vi "Optimize Extended Rosenbrock.vi"() -> ()   [LabVIEW 2016]
doc: "This VI shows an example of using the Unconstrained Optimization VI. The VI uses the Extended Rosenbrock Function VI to create an objective function. The VI then passes this function to the Unconstrained Optimization VI."
uses:
  <vilib>/Math Plots/3D Math Plots/3D Surface/3D Surface XCtrl/3D Surface.xctl
  <vilib>/Math Plots/3D Math Plots/3D Plot/3D Plot/Typedef/Color Ramp Cluster.ctl
  <vilib>/Analysis/1siggen.llb/Ramp Pattern by Samples.vi
  <vilib>/Math Plots/3D Math Plots/3D Surface/3D Surface Datatype/Public/Plot Helper (Vector).vi
  <vilib>/gmath/NumericalOptimization/Quasi Newton.vi
  <vilib>/gmath/NumericalOptimization/Conjugate Gradient.vi
  <vilib>/gmath/NumericalOptimization/Downhill Simplex.vi
  <vilib>/gmath/NI_Gmath.lvlib
  <vilib>/Analysis/NI_AALBase.lvlib
  <vilib>/Math Plots/3D Math Plots/3D Surface/3D Surface Datatype/3D Surface Datatype.lvclass
  <vilib>/Math Plots/3D Math Plots/3D Plot/3D Plot/3D Plot.lvclass
panel:
  in  "Conjugate gradient settings":T1={"gradient method"=enum."Polak-Ribiere", "line minimization"=enum."with derivatives"}
  in  "Stopping criteria":T2={"function tolerance"=1e-08, "parameter tolerance"=1e-10, "max iterations"=10000, "max function calls"=10000, "gradient tolerance"=-1.0, "max time (sec)"=-1.0}
  in  "Optimization Method":T3(ring)
  in  "Animate solution?":bool=TRUE
  out "Intensity Graph":dbl[][](graph)
  out "3D Surface":refnum<class "3D Plot Datatype.lvclass">[](xcontrol)
  out "Number of function evaluations":i32
  out "Minimum Value":dbl
  out "Minimum":dbl[](array[numeric])
  in  "Start":dbl[](array[numeric])=[-1.2, 2.0]
  # "Overview: Demonstrates the use of the Unconstrained Optimization VI.\nRequirements: LabVIEW Full Development System\nInstructions:\n1. Select an Optimization Method and Start position of the optimization.\n2. Run the VI and, if you have Animate Solution? set to TRUE, you can see the path of the solver on the Intensity Graph. If the solver can find the solution, you would be able to see the minimum at [1,1]. Try to run the VI again with Animate Solution? set to FALSE to observe the speed of the algorithm.\n3. Add two more points to the Start array making [-1.2, 2, -1.2, 2]. Although the graph will only show the first two variables, the Minimum array will show more points, all at 1."
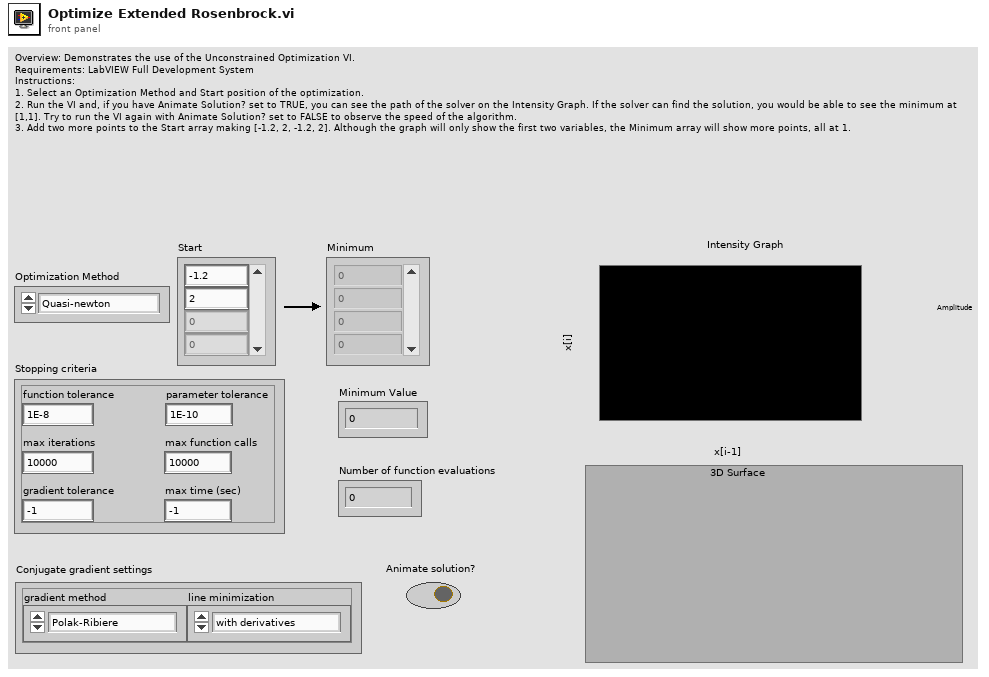
[diagram p1: front panel]
types:
  T1 = cluster{"gradient method":enum16{"Fletcher-Reeves", "Polak-Ribiere"}, "line minimization":enum16{"without derivatives", "with derivatives"}}
  T2 = cluster{"function tolerance":dbl, "parameter tolerance":dbl, "max iterations":i32, "max function calls":i32, "gradient tolerance":dbl, "max time (sec)":dbl}
  T3 = enum16{"Quasi-newton", "Conjugate Gradient", "Downhill Simplex"}
  T4 = enum16{"None", "Shaded", "Color spectrum", "Grey scale", "Custom"}
  T5 = typedef "3D Plot.lvclass/Color Ramp Cluster.ctl" = cluster{"Color Ramp Style":enum16{"None", "Shaded", "Color spectrum", "Grey scale", "Custom"}, "Color Ramp Array":u32[], "Color Ramp Index":i32[], "Interpolate?":bool, "Logarithm?":bool}
  T6 = cluster{"c":dbl, "Intensity Graph":refnum<vi>, "animate?":bool}
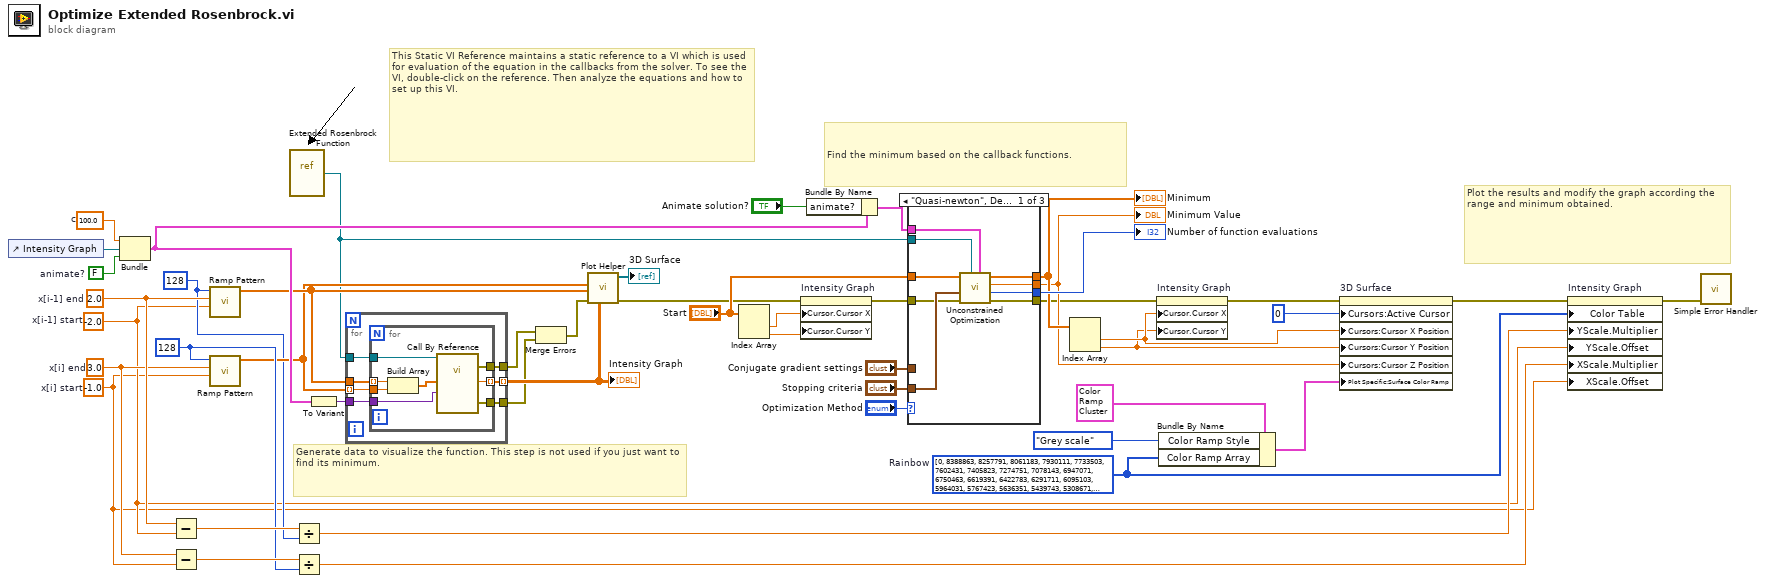
[diagram p0: block diagram]
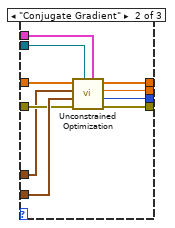
[diagram p2: hidden frame]
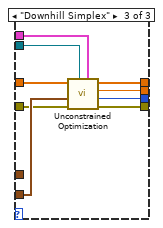
[diagram p3: hidden frame]
diagram:
  w33 = 100.0  # c
  w18 = 128 ("samples")
  w32 = FALSE  # animate?
  w41 = u32[] [0, 8388863, 8257791, 8061183, 7930111, 7733503, 7602431, 7405823, 7274751, 7078143, 6947071, 6750463, 6619391, 6422783, 6291711, 6095103, 5964031, 5767423, 5636351, 5439743, 5308671, 5112063, 4980991, 4784383, 4653311, 4456703, 4325631, 4129023, 3932415, 3801343, 3604735, 3473663, 3277055, 3145983, 2949375, 2818303, 2621695, 2490623, 2294015, 2162943, 1966335, 1835263, 1638655, 1507583, 1310975, 1179903, 983295, 852223, 655615, 524543, 327935, 196863, 511, 1791, 3071, 4351, 5631, 6911, 8191, 9471, 10751, 12031, 13311, 14591, 15871, 17151, 18431, 19711, 20991, 22271, 23551, 24831, 26111, 27391, 28671, 29951, 31231, 32511, 33791, 35071, 36351, 37631, 38911, 40191, 41471, 42751, 44031, 45311, 46591, 47871, 49151, 50431, 51711, 52991, 54271, 55551, 56831, 58111, 59391, 60671, 61951, 63231, 64511, 65532, 65527, 65522, 65517, 65512, 65507, 65502, 65497, 65492, 65487, 65482, 65477, 65472, 65467, 65462, 65457, 65452, 65447, 65442, 65437, 65432, 65427, 65422, 65417, 65412, 65407, 65402, 65397, 65392, 65387, 65382, 65377, 65372, 65367, 65362, 65357, 65352, 65347, 65342, 65337, 65332, 65327, 65322, 65317, 65312, 65307, 65302, 65297, 65292, 65287, 65282, 261888, 589568, 917248, 1244928, 1572608, 1900288, 2227968, 2555648, 2883328, 3211008, 3538688, 3866368, 4194048, 4521728, 4849408, 5177088, 5504768, 5832448, 6160128, 6487808, 6815488, 7143168, 7470848, 7798528, 8126208, 8453888, 8781568, 9109248, 9436928, 9764608, 10092288, 10419968, 10747648, 11075328, 11403008, 11730688, 12058368, 12386048, 12713728, 13041408, 13369088, 13696768, 14024448, 14352128, 14679808, 15007488, 15335168, 15662848, 15990528, 16318208, 16645888, 16775936, 16774656, 16773376, 16772096, 16770816, 16769536, 16768256, 16766976, 16765696, 16764416, 16763136, 16761856, 16760576, 16759296, 16758016, 16756736, 16755456, 16754176, 16752896, 16751616, 16750336, 16749056, 16747776, 16746496, 16745216, 16743936, 16742656, 16741376, 16740096, 16738816, 16737536, 16736256, 16734976, 16733696, 16732416, 16731136, 16729856, 16728576, 16727296, 16726016, 16724736, 16723456, 16722176, 16720896, 16719616, 16718336, 16717056, 16715776, 16714496, 16713216, 16711680]  # Rainbow
  w12 = 128 ("samples")
  w11 = -2.0  # x[i-1] start
  w39 = 2.0  # x[i-1] end
  w10 = -1.0  # x[i] start
  w36 = 3.0  # x[i] end
  # "Plot the results and modify the graph according the range and minimum obtained."
  # "Find the minimum based on the callback functions."
  # "Generate data to visualize the function. This step is not used if you just want to find its minimum."
  # "This Static VI Reference maintains a static reference to a VI which is used for evaluation of the equation in the callbacks from the solver. To see the VI, double-click on the reference. Then analyze the equations and how to set up this VI."
  n1 = control-ref of="Intensity Graph"() -> (w34:refnum<vi>)
  n2 = Bundle("c"=w33, "Intensity Graph"=w34, "animate?"=w32) -> (w31:T6)  [unwired: 1 in]
  n3 = Subtract(x=w39, y=w11) -> (x-y=w38:dbl)
  n4 = Subtract(x=w36, y=w10) -> (x-y=w37:dbl)
  n5 = call-poly <vilib>:"Ramp Pattern.vi"("start"=w11, "end"=w39, "samples"=w12) -> ("Ramp Pattern"=w19:dbl[])  [unwired: 7 in, 1 out]
  n6 = call-poly <vilib>:"Ramp Pattern.vi"("start"=w10, "end"=w36, "samples"=w18) -> ("Ramp Pattern"=w17:dbl[])  [unwired: 7 in, 1 out]
  n7 = vi-ref "Extended Rosenbrock Function.vi"() -> (w15:refnum<vi>)
  n8 = Divide(x=w38, y=w12) -> (x/y=w40:dbl)
  n9 = Divide(x=w37, y=w18) -> (x/y=w13:dbl)
  n10 = To Variant(anything=w31) -> (Variant=w44:variant)
  n11 = for {
    tunnel: [w54] -> w24 mode=indexing
    tunnel: w19 -> [w53]
    tunnel: w17 -> [w52] mode=indexing
    tunnel: w44 -> [w51]
    tunnel: [w50] -> w2
    tunnel: w15 -> [w49]
    tunnel: [w48] -> w3
    n12 = for {
      tunnel: [w62] -> w54 mode=indexing
      tunnel: w53 -> [w58] mode=indexing
      tunnel: w52 -> [w59]
      tunnel: w51 -> [w60]
      tunnel: [w57] -> w50
      tunnel: w49 -> [w56]
      tunnel: [w55] -> w48
      n13 = Build Array(w58, w59) -> (w61:dbl[])
      n14 = call-by-ref "?"(reference=w56, "data"=w60, "X"=w61) -> (error out=w55:errorcluster, 0:"error out"=w57:errorcluster, "f(X)"=w62:dbl)  [unwired: 2 in, 2 out]
    }
  }
  "Intensity Graph" <- w24
  n15 = Merge Errors(w3, w2) -> (w1:errorcluster)
  n16 = call-poly <vilib>:"Plot Helper.vi"("z matrix"=w24, "error in (no error)"=w1, "y vector"=w19, "x vector"=w17) -> ("error out"=w5:errorcluster, "3D Plot lvclass Array out"=→"3D Surface":refnum<class "3D Plot Datatype.lvclass">[])  [unwired: 2 in, 4 out]
  n17 = Index Array(array="Start") -> (element #1=w7:dbl, element #2=w6:dbl)  [unwired: 2 in]
  n18 = property on="Intensity Graph" class="IntGraph (strict)"(error in=w5, "Cursor.Cursor X"=w7, "Cursor.Cursor Y"=w6) -> (error out=w4:errorcluster)  [unwired: 1 in, 1 out]
  n19 = Bundle By Name(cluster=w31, "animate?"="Animate solution?") -> (w30:T6)
  n20 = case shown="\"Quasi-newton\", Default" "Optimization Method" {
    tunnel: "Start" -> [w71 w81 w90]
    tunnel: [w70 w80 w89] -> w47
    tunnel: "Stopping criteria" -> [w69 w79 w88]
    tunnel: w4 -> [w68 w78 w87]
    tunnel: [w67 w77 w86] -> w35
    tunnel: w30 -> [w66 w76 w85]
    tunnel: [w65 w75 w84] -> w25
    tunnel: [w64 w74 w83] -> w22
    tunnel: w15 -> [w63 w73 w82]
    tunnel: "Conjugate gradient settings" -> [_ w72 _]
    frame "Quasi-newton", Default {
      n21 = call-poly <vilib>:"Unconstrained Optimization.vi"("function data"=w66, "objective function"=w63, "error in (no error)"=w68, "stopping criteria"=w69, "start"=w71) -> ("error out"=w64:errorcluster, "number of function evaluations"=w70:i32, "f(minimum)"=w65:dbl, "minimum"=w67:dbl[])  [unwired: 3 in]
    }
    frame "Conjugate Gradient" {
      n22 = call-poly <vilib>:"Unconstrained Optimization.vi"("function data"=w76, "objective function"=w73, "error in (no error)"=w78, "stopping criteria"=w79, "conjugate gradient settings"=w72, "start"=w81) -> ("error out"=w74:errorcluster, "number of function evaluations"=w80:i32, "f(minimum)"=w75:dbl, "minimum"=w77:dbl[])  [unwired: 2 in]
    }
    frame "Downhill Simplex" {
      n23 = call-poly <vilib>:"Unconstrained Optimization.vi"("function data"=w85, "objective function"=w82, "error in (no error)"=w87, "stopping criteria"=w88, "start"=w90) -> ("error out"=w83:errorcluster, "number of function evaluations"=w89:i32, "f(minimum)"=w84:dbl, "minimum"=w86:dbl[])  [unwired: 3 in]
    }
  }
  "Minimum" <- w35
  "Minimum Value" <- w25
  "Number of function evaluations" <- w47
  n24 = Index Array(array=w35) -> (element #1=w28:dbl, element #2=w27:dbl)  [unwired: 2 in]
  n25 = property on="Intensity Graph" class="IntGraph (strict)"(error in=w22, "Cursor.Cursor X"=w28, "Cursor.Cursor Y"=w27) -> (error out=w21:errorcluster)  [unwired: 1 in, 1 out]
  n26 = Bundle By Name(cluster=T5 {"Color Ramp Style"=enum."None", "Color Ramp Array"=[16711934, 393471, 57855, 4390754, 16449346, 16744722, 16711680], "Color Ramp Index"=[45, 91, 133, 175, 219, 255], "Interpolate?"=FALSE, "Logarithm?"=FALSE} ("Plot Specific:Surface:Surface Color Ramp"), "Color Ramp Style"=T4."Grey scale", "Color Ramp Array"=w41) -> (w20:T5)
  n27 = property on="3D Surface" class="3D Surface (strict)"(error in=w21, "Cursors:Active Cursor"=0, "Cursors:Cursor X Position"=w28, "Cursors:Cursor Y Position"=w27, "Cursors:Cursor Z Position"=w25, "Plot Specific:Surface Color Ramp"=w20) -> (error out=w23:errorcluster)  [unwired: 1 in, 1 out]
  n28 = property on="Intensity Graph" class="IntGraph (strict)"(error in=w23, "Color Table"=w41, "YScale.Multiplier"=w40, "YScale.Offset"=w11, "XScale.Multiplier"=w13, "XScale.Offset"=w10) -> (error out=w16:errorcluster)  [unwired: 1 in, 1 out]
  n29 = call <vilib>:"Simple Error Handler.vi"("error in (no error)"=w16) -> ()  [unwired: 4 in, 5 out]
